vi "Obtain Request Events.vi"(8 "error in":errorcluster, 10 "Create New? (F)":bool) -> (0 "error out":errorcluster, 2 "GUI Request Events":T1)   [LabVIEW 2024, in "GUI.lvlib"]
doc: "This VI Obtains/Creates the Requests events that will be used for other modules to communicate with the module that owns this VI. These Requests events will be accessed only via Public API methods for this module.\n\n<b>NOTE</b>: The contents of this VI are automatically generated and modified by the <b>Tools > DQMH Consortium > DQMH</b> utilities. Consider using those utilities instead of making your own modifications to this VI.\n_____\nBased on DQMH Dev Tools: Project Template 7.1.0.1503."
uses:
  GUI.lvlib
  Request Events--cluster.ctl
  Stop Argument--cluster.ctl
  Show Panel Argument--cluster.ctl
  Hide Panel Argument--cluster.ctl
  Get Module Execution Status Argument--cluster.ctl
  Show Diagram Argument--cluster.ctl
  login Argument--cluster.ctl
  DB/Controls/Login info.ctl
  DB/Controls/User level.ctl
  login_ Argument--cluster.ctl
  logout Argument--cluster.ctl
  Load settings Argument--cluster.ctl
  Controls/Settings.ctl
  update serials array Argument--cluster.ctl
  update parent Argument--cluster.ctl
  update HW status indicator Argument--cluster.ctl
  Controls/HW Modules.ctl
panel:
  # "NOTE: The contents of this VI are automatically generated and modified by the Tools > DQMH Consortium > DQMH utilities. Consider using those utilities instead of making your own modifications to this VI."
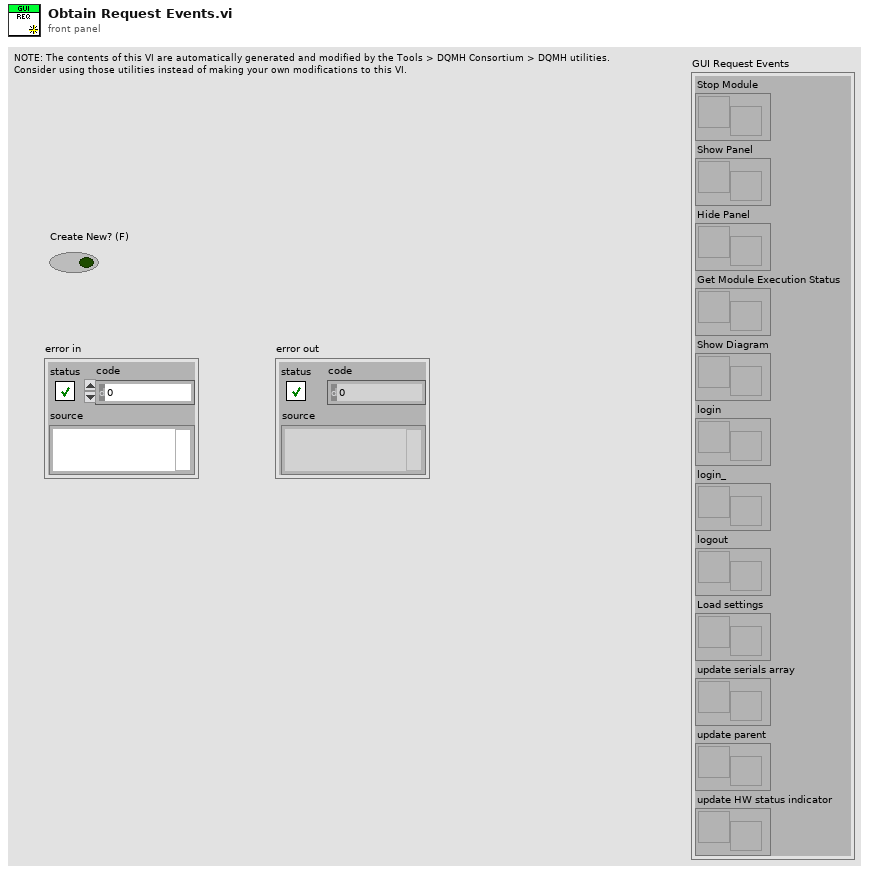
[diagram p1: front panel]
types:
  T1 = typedef "GUI.lvlib/Request Events--cluster.ctl" = cluster{"Stop Module":refnum<user-event>, "Show Panel":refnum<user-event>, "Hide Panel":refnum<user-event>, "Get Module Execution Status":refnum<user-event>, "Show Diagram":refnum<user-event>, "login":refnum<user-event>, "login_":refnum<user-event>, "logout":refnum<user-event>, "Load settings":refnum<user-event>, "update serials array":refnum<user-event>, "update parent":refnum<user-event>, "update HW status indicator":refnum<user-event>}
  T2 = typedef "GUI.lvlib/update HW status indicator Argument--cluster.ctl" = cluster{"HW Module":T3, "Status":bool}
  T3 = typedef "HW Modules.ctl" = string
  T4 = typedef "GUI.lvlib/update parent Argument--cluster.ctl" = cluster{"Parent":string, "level":dbl}
  T5 = typedef "GUI.lvlib/update serials array Argument--cluster.ctl" = cluster{"serial array":string[], "level":dbl}
  T6 = typedef "GUI.lvlib/Load settings Argument--cluster.ctl" = cluster{"Settings":T7, "reconnect":bool}
  T7 = typedef "Settings.ctl" = cluster{"Camera 1 IP":string, "Camera 2 IP":string, "Printer 1 IP":string, "Printer 2 IP":string, "Level 2 Scanner COM":refnum<visa-resource-name>, "PLC Port":dbl, "PLC IP":string, "Handheld Scanner COM":refnum<visa-resource-name>, "Printer2 Port":dbl, "Cam1 send port ":dbl, "Cam1 recv port":dbl, "Cam2 send port":dbl, "Cam recv port":dbl, "Printer1 Port":dbl}
  T8 = typedef "GUI.lvlib/logout Argument--cluster.ctl" = cluster{"Boolean":bool}
  T9 = typedef "GUI.lvlib/login_ Argument--cluster.ctl" = cluster{"Login info":T10}
  T10 = typedef "Login info.ctl" = cluster{"User Name":string, "User level":T11}
  T11 = typedef "User level.ctl" = enum16{"Operator", "Admin"}
  T12 = typedef "GUI.lvlib/login Argument--cluster.ctl" = cluster{"Login info":T10}
  T13 = typedef "GUI.lvlib/Hide Panel Argument--cluster.ctl" = cluster{"Hide Panel?":bool}
  T14 = typedef "GUI.lvlib/Show Panel Argument--cluster.ctl" = cluster{"Show Panel?":bool}
  T15 = typedef "GUI.lvlib/Show Diagram Argument--cluster.ctl" = cluster{"Debug?":bool}
  T16 = typedef "GUI.lvlib/Get Module Execution Status Argument--cluster.ctl" = cluster{"Running?":bool}
  T17 = typedef "GUI.lvlib/Stop Argument--cluster.ctl" = cluster{"Origin":string, "Exit via Stop Module Req?":bool, "Wait for Module to stop?":bool}
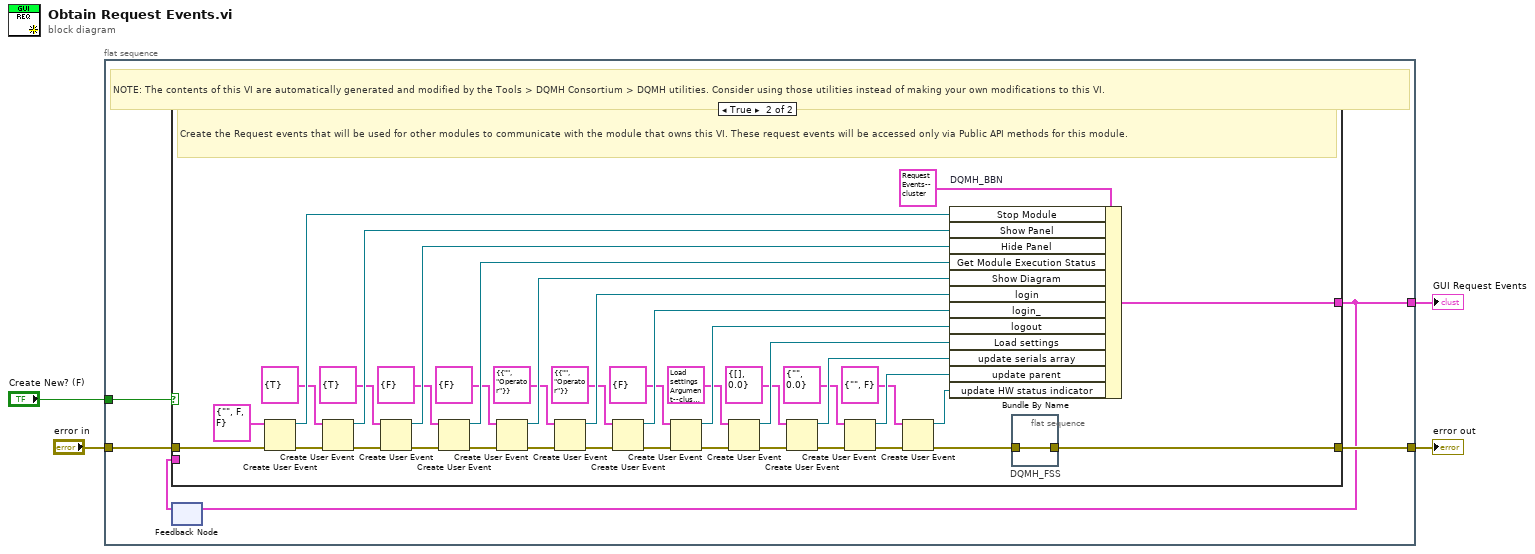
[diagram p0: block diagram]
diagram:
  n1 = flat-sequence {
    tunnel: [w9] -> w4
    tunnel: "error in" -> [w8]
    tunnel: [w6] -> w2
    tunnel: "Create New? (F)" -> [w5]
    frame #0 {
      # "NOTE: The contents of this VI are automatically generated and modified by the Tools > DQMH Consortium > DQMH utilities. Consider using those utilities instead of making your own modifications to this VI."
      n2 = feedback #1() -> (w7:T1)  [unwired: 1 in]
      n3 = case shown="True" w5 {
        tunnel: [w10 w41] -> w9
        tunnel: w8 -> [w10 w51]
        tunnel: [w11 w48] -> w6
        tunnel: w7 -> [w11 _]
        frame False {
          # "Obtain the Request events that were created in a previous call to this VI."
        }
        frame True {
          # "Create the Request events that will be used for other modules to communicate with the module that owns this VI. These request events will be accessed only via Public API methods for this module."
          n4 = Create User Event(user event datatype=T17 {"Origin"="", "Exit via Stop Module Req?"=FALSE, "Wait for Module to stop?"=FALSE} ("Stop Argument"), error in=w51) -> (user event=w49:refnum<user-event>, error out=w46:errorcluster)
          n5 = Create User Event(user event datatype=T14 {"Show Panel?"=TRUE} ("Show Panel Argument"), error in=w46) -> (user event=w45:refnum<user-event>, error out=w44:errorcluster)
          n6 = Create User Event(user event datatype=T13 {"Hide Panel?"=TRUE} ("Hide Panel Argument"), error in=w44) -> (user event=w43:refnum<user-event>, error out=w42:errorcluster)
          n7 = Create User Event(user event datatype=T16 {"Running?"=FALSE} ("Get Module Execution Status Argument"), error in=w42) -> (user event=w39:refnum<user-event>, error out=w40:errorcluster)
          n8 = Create User Event(user event datatype=T15 {"Debug?"=FALSE} ("Show Diagram Argument"), error in=w40) -> (user event=w36:refnum<user-event>, error out=w37:errorcluster)
          n9 = Create User Event(user event datatype=T12 {"Login info"={"User Name"="", "User level"=enum."Operator"}} ("login Argument"), error in=w37) -> (user event=w31:refnum<user-event>, error out=w32:errorcluster)
          n10 = Create User Event(user event datatype=T9 {"Login info"={"User Name"="", "User level"=enum."Operator"}} ("login_ Argument"), error in=w32) -> (user event=w28:refnum<user-event>, error out=w29:errorcluster)
          n11 = Create User Event(user event datatype=T8 {"Boolean"=FALSE} ("logout Argument"), error in=w29) -> (user event=w25:refnum<user-event>, error out=w26:errorcluster)
          n12 = Create User Event(user event datatype=T6 {"Settings"={"Camera 1 IP"="", "Camera 2 IP"="", "Printer 1 IP"="", "Printer 2 IP"="", "Level 2 Scanner COM"="", "PLC Port"=0.0, "PLC IP"="", "Handheld Scanner COM"="", "Printer2 Port"=0.0, "Cam1 send port "=0.0, "Cam1 recv port"=0.0, "Cam2 send port"=0.0, "Cam recv port"=0.0, "Printer1 Port"=0.0}, "reconnect"=FALSE} ("Load settings Argument"), error in=w26) -> (user event=w22:refnum<user-event>, error out=w23:errorcluster)
          n13 = Create User Event(user event datatype=T5 {"serial array"=[], "level"=0.0} ("update serials array Argument"), error in=w23) -> (user event=w19:refnum<user-event>, error out=w20:errorcluster)
          n14 = Create User Event(user event datatype=T4 {"Parent"="", "level"=0.0} ("update parent Argument"), error in=w20) -> (user event=w16:refnum<user-event>, error out=w17:errorcluster)
          n15 = Create User Event(user event datatype=T2 {"HW Module"="", "Status"=FALSE} ("update HW status indicator Argument"), error in=w17) -> (user event=w13:refnum<user-event>, error out=w14:errorcluster)
          n16 = Bundle By Name "DQMH_BBN"(cluster=T1 {"Stop Module"=refnum, "Show Panel"=refnum, "Hide Panel"=refnum, "Get Module Execution Status"=refnum, "Show Diagram"=refnum, "login"=refnum, "login_"=refnum, "logout"=refnum, "Load settings"=refnum, "update serials array"=refnum, "update parent"=refnum, "update HW status indicator"=refnum} ("output cluster"), "Stop Module"=w49, "Show Panel"=w45, "Hide Panel"=w43, "Get Module Execution Status"=w39, "Show Diagram"=w36, "login"=w31, "login_"=w28, "logout"=w25, "Load settings"=w22, "update serials array"=w19, "update parent"=w16, "update HW status indicator"=w13) -> (w48:T1)
          n17 = flat-sequence "DQMH_FSS" {
            tunnel: w14 -> [w52]
            tunnel: [w52] -> w41
            frame #0 {
            }
          }
        }
      }
      n18 = feedback-in #1(w6) -> ()
    }
  }
  "GUI Request Events" <- w2
  "error out" <- w4
